vi "Parse Option String.vi"(0 "option string":string, 11 "error in":errorcluster) -> (4 "option name/value pairs":cluster{"option":string, "value":string}[](array[cluster]), 15 "error out":errorcluster)   [LabVIEW 2019]
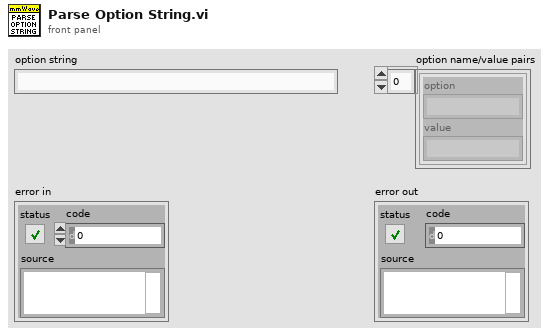
[diagram p1: front panel]
types:
  T1 = cluster{"trimmed string":string, "trimmed string":string}
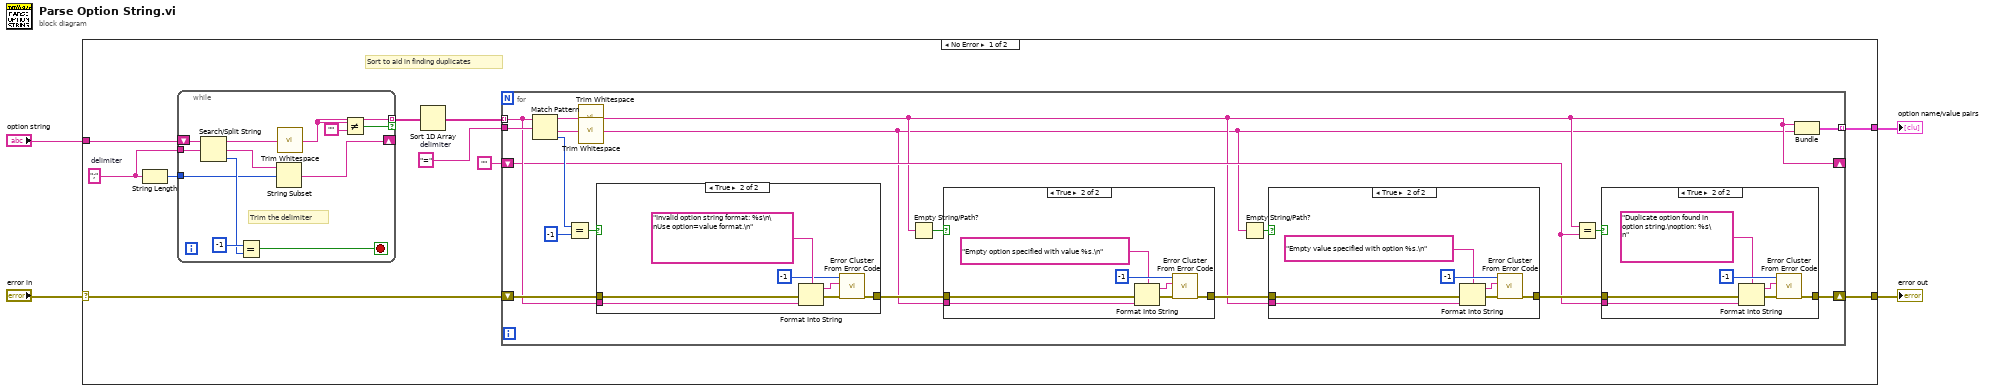
[diagram p0: block diagram]
diagram:
  n1 = case shown="No Error" "error in" {
    selector: "error in" -> [w7 w78]
    tunnel: "option string" -> [w14 _]
    tunnel: [w6 w78] -> w3
    tunnel: [w5 _] -> w1
    frame No Error {
      w11 = "="  # delimiter
      w13 = ";"  # delimiter
      # "Sort to aid in finding duplicates"
      n2 = String Length(string=w13) -> (length=w12:i32)
      n3 = while {
        shift-right: [w74] -> _
        shift-left: w14 -> [w77]
        tunnel: w13 -> [w76]
        tunnel: [w68] -> w9 mode=indexing if=w69
        tunnel: w12 -> [w71]
        stop <- w66 stop-if-true
        # "Trim the delimiter"
        n4 = Search/Split String(string=w77, search string/char (-)=w76) -> (substring before match=w70:string, match + rest of string=w75:string, offset of match=w72:i32)  [unwired: 1 in]
        n5 = Equal?(x=-1 ("y"), y=w72) -> (x = y?=w66:bool)
        n6 = String Subset(string=w75, offset (0)=w71) -> (substring=w74:string)  [unwired: 1 in]
        n7 = call <vilib>:"Trim Whitespace.vi"("string"=w70) -> ("trimmed string"=w68:string)  [unwired: 1 in]
        n8 = Not Equal?(x=w68, y="") -> (x != y?=w69:bool)
      }
      n9 = Sort 1D Array(array=w9) -> (sorted array=w10:string[])
      n10 = for {
        tunnel: w10 -> [w28] mode=indexing
        tunnel: w11 -> [w30]
        shift-right: [w19] -> w6
        shift-left: w7 -> [w29]
        shift-right: [w17] -> _
        shift-left: "" -> [w18]
        tunnel: [w15] -> w5 mode=indexing
        n11 = Match Pattern(string=w28, regular expression=w30) -> (before substring=w23:string, after substring=w24:string, offset past match=w33:i32)  [unwired: 1 in, 1 out]
        n12 = Equal?(x=w33, y=-1) -> (x = y?=w31:bool)
        n13 = call <vilib>:"Trim Whitespace.vi"("string"=w23) -> ("trimmed string"=w17:string)  [unwired: 1 in]
        n14 = call <vilib>:"Trim Whitespace.vi"("string"=w24) -> ("trimmed string"=w16:string)  [unwired: 1 in]
        n15 = case shown="True" w31 {
          tunnel: w28 -> [_ w64]
          tunnel: [w58 w61] -> w22
          tunnel: w29 -> [w58 w60]
          frame False {
          }
          frame True {
            n16 = Format Into String(format string="Invalid option string format: %s\n\nUse option=value format.\n" ("error message (\"\")"), error in=w60, w64) -> (resulting string=w63:string, error out=w59:errorcluster)  [unwired: 1 in]
            n17 = call <vilib>:"Error Cluster From Error Code.vi"("error in (no error)"=w59, "error message (\"\")"=w63, "error code (0)"=-1) -> ("error out"=w61:errorcluster)  [unwired: 6 in]
          }
        }
        n18 = Empty String/Path?(string/path=w17) -> (empty?=w25:bool)
        n19 = case shown="True" w25 {
          tunnel: w22 -> [w42 w47]
          tunnel: [w42 w49] -> w26
          tunnel: w16 -> [_ w44]
          frame False {
          }
          frame True {
            n20 = Format Into String(format string="Empty option specified with value %s.\n" ("error message (\"\")"), error in=w47, w44) -> (resulting string=w45:string, error out=w46:errorcluster)  [unwired: 1 in]
            n21 = call <vilib>:"Error Cluster From Error Code.vi"("error in (no error)"=w46, "error message (\"\")"=w45, "error code (0)"=-1) -> ("error out"=w49:errorcluster)  [unwired: 6 in]
          }
        }
        n22 = Empty String/Path?(string/path=w16) -> (empty?=w27:bool)
        n23 = case shown="True" w27 {
          tunnel: w26 -> [w50 w55]
          tunnel: [w50 w57] -> w20
          tunnel: w17 -> [_ w51]
          frame False {
          }
          frame True {
            n24 = Format Into String(format string="Empty value specified with option %s.\n" ("error message (\"\")"), error in=w55, w51) -> (resulting string=w53:string, error out=w54:errorcluster)  [unwired: 1 in]
            n25 = call <vilib>:"Error Cluster From Error Code.vi"("error in (no error)"=w54, "error message (\"\")"=w53, "error code (0)"=-1) -> ("error out"=w57:errorcluster)  [unwired: 6 in]
          }
        }
        n26 = Equal?(x=w17, y=w18) -> (x = y?=w21:bool)
        n27 = case shown="True" w21 {
          tunnel: w20 -> [w34 w38]
          tunnel: [w34 w41] -> w19
          tunnel: w18 -> [_ w39]
          frame False {
          }
          frame True {
            n28 = Format Into String(format string="Duplicate option found in option string.\noption: %s\n" ("error message (\"\")"), error in=w38, w39) -> (resulting string=w36:string, error out=w37:errorcluster)  [unwired: 1 in]
            n29 = call <vilib>:"Error Cluster From Error Code.vi"("error in (no error)"=w37, "error message (\"\")"=w36, "error code (0)"=-1) -> ("error out"=w41:errorcluster)  [unwired: 6 in]
          }
        }
        n30 = Bundle("trimmed string"=w17, "trimmed string"=w16) -> (w15:T1)  [unwired: 1 in]
      }
    }
    frame Error {
    }
  }
  "error out" <- w3
  "option name/value pairs" <- w1
